vi "passFail.vi"(6 "TacticIndex":dbl, 8 "error in (no error)":errorcluster, 9 "Offensive Robots":refnum<class "Robot.lvclass">[](array[class]), 10 "Ball":refnum<class "Ball.lvclass">, 11 "Play in":refnum<class "Play.lvclass">) -> (0 "error out":errorcluster, 2 "PassFail?":bool, 3 "Play out":refnum<class "Play.lvclass">)   [LabVIEW 2023, in "Play.lvclass"]
uses:
  Play.lvclass
  Ball_class/Ball.lvclass
  Robot_class/Robot.lvclass
  Utilities_class/Utilities.lvclass
  Ball_class/Ball.lvclass/Ball.ctl
  Ball_class/Read v_x.vi
  Ball_class/Read v_y.vi
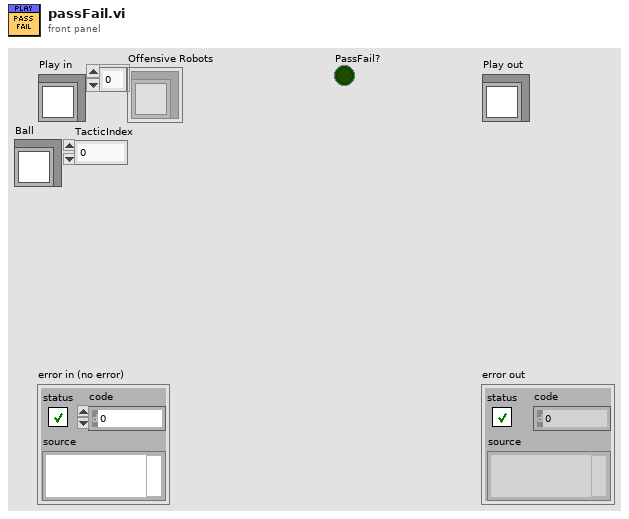
[diagram p1: front panel]
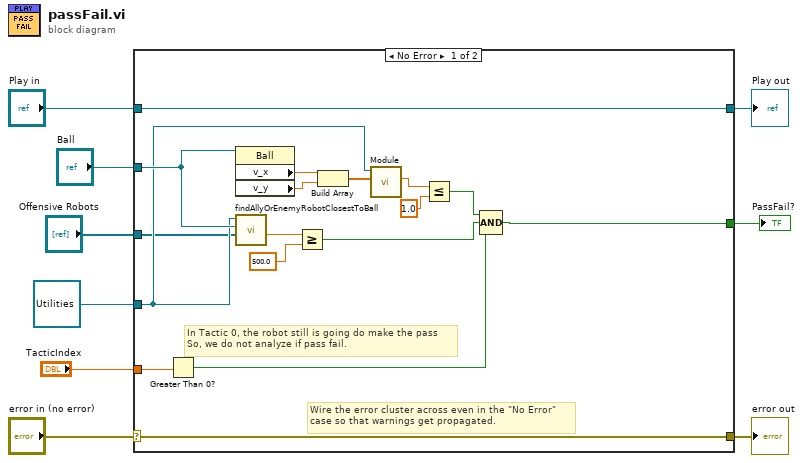
[diagram p0: block diagram]
diagram:
  n1 = case shown="No Error" "error in (no error)" {
    selector: "error in (no error)" -> [w25 w28]
    tunnel: [w25 w28] -> w8
    tunnel: [w26 w27] -> w6
    tunnel: "Play in" -> [w26 w27]
    tunnel: "Ball" -> [w24 _]
    tunnel: "Offensive Robots" -> [w12 _]
    tunnel: [w14 _] -> w3
    tunnel: refnum<class "Utilities.lvclass"> refnum ("Utilities.lvclass") -> [w13 _]
    tunnel: "TacticIndex" -> [w11 _]
    frame No Error {
      # "In Tactic 0, the robot still is going do make the pass\nSo, we do not analyze if pass fail."
      # "Wire the error cluster across even in the \"No Error\"\ncase so that warnings get propagated."
      n2 = Greater Than 0?(x=w11) -> (x > 0?=w10:bool)
      n3 = property class="Ball"(reference=w24) -> ("v_x"=w23:dbl, "v_y"=w22:dbl)  [unwired: 1 in, 2 out]
      n4 = call "findAllyOrEnemyRobotClosestToBall.vi"("Ally/Enemy Robots"=w12, "Ball"=w24, "Utilities in"=w13) -> ("Robot distance to ball"=w18:dbl)  [unwired: 4 in, 4 out]
      n5 = Greater Or Equal?(x=w18, y=500.0) -> (x >= y?=w15:bool)
      n6 = Build Array(w23, w22) -> (w21:dbl[])
      n7 = call "Module.vi"("2D vector"=w21, "Utilities in"=w13) -> ("Modulo"=w20:dbl)  [unwired: 7 in, 2 out]
      n8 = Less Or Equal?(x=w20, y=1.0) -> (x <= y?=w16:bool)
      n9 = Compound Arithmetic op=AND(w16, w15, w10) -> (w14:bool)
    }
    frame Error {
    }
  }
  "error out" <- w8
  "Play out" <- w6
  "PassFail?" <- w3
